vi "data更新获取索引操作函数.vi"(8 "error in (no error)":errorcluster, 9 "当前操作行":i32, 10 "当前_datetime":string, 11 "缓存操作选项":T1) -> (0 "error out":errorcluster, 3 "Data_CT索引操作缓存":T2)   [LabVIEW 2017]
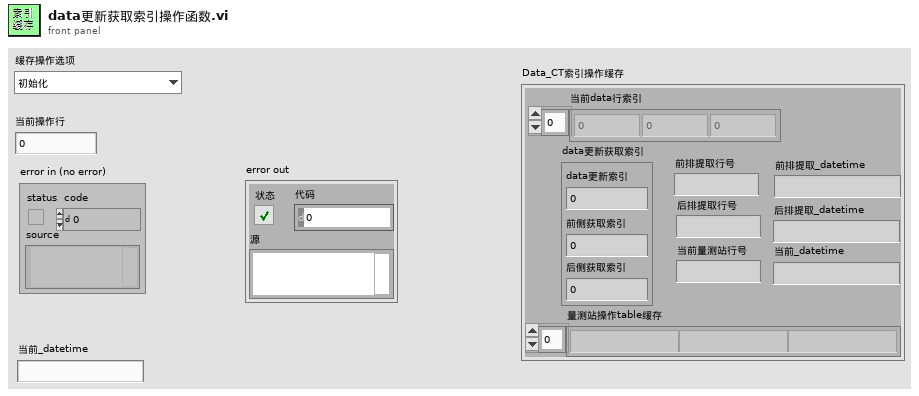
[diagram p1: front panel]
types:
  T1 = typedef "缓存操作选项.ctl" = enum16{"初始化", "量测缓存写入", "前侧获取索引", "后侧获取索引", "前侧更新索引", "后侧更新索引", "获取寄存器"}
  T2 = typedef "Data_CT索引操作缓存.ctl" = cluster{"当前data行索引":i32[], "data更新获取索引":T3, "前排提取行号":string, "后排提取行号":string, "当前量测站行号":string, "当前_datetime":string, "量测站操作table缓存":string[], "前排提取_datetime":string, "后排提取_datetime":string}
  T3 = typedef "data更新获取索引.ctl" = cluster{"data更新索引":i32, "前侧获取索引":i32, "后侧获取索引":i32}
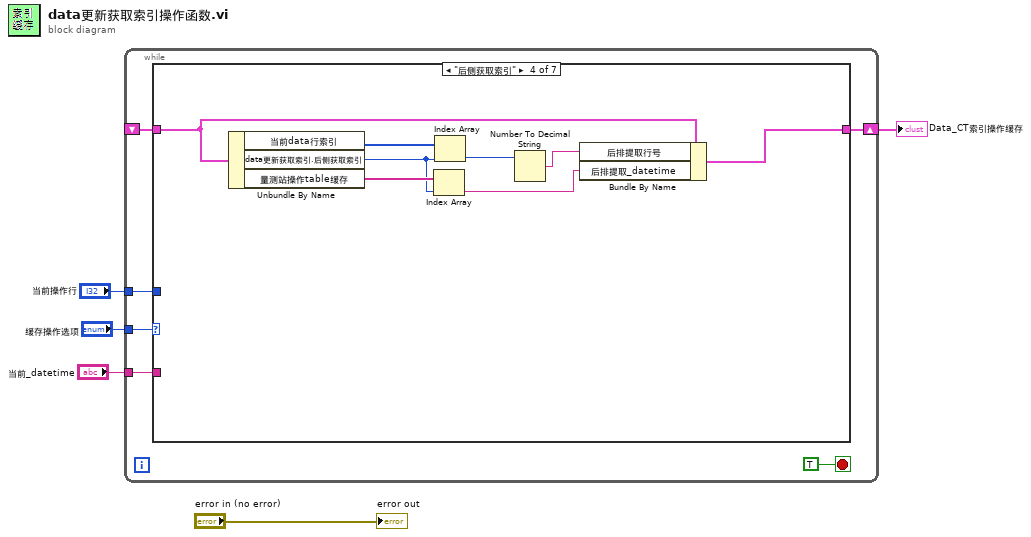
[diagram p0: block diagram]
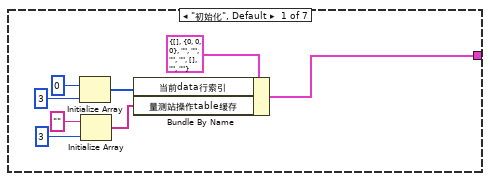
[diagram p2: hidden frame]
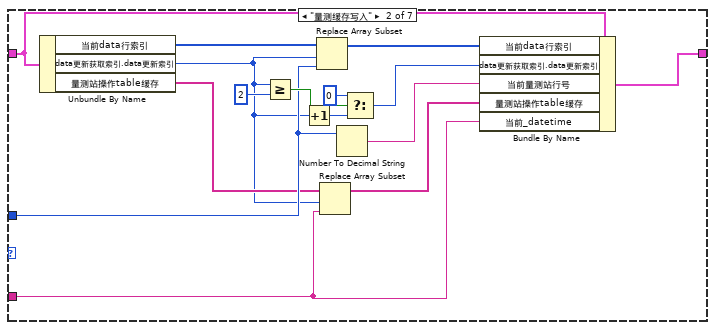
[diagram p3: hidden frame]
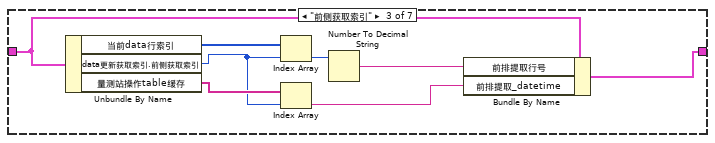
[diagram p4: hidden frame]
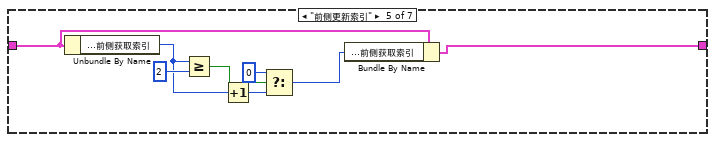
[diagram p5: hidden frame]
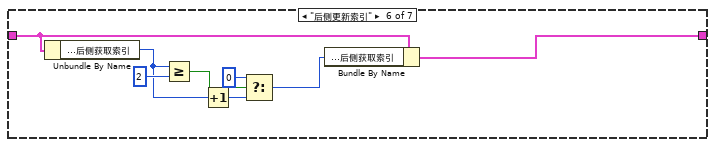
[diagram p6: hidden frame]
diagram:
  n1 = while {
    tunnel: "缓存操作选项" -> [w11]
    shift-right: [w9] -> w4
    shift-left: _ -> [w8]
    tunnel: "当前操作行" -> [w7]
    tunnel: "当前_datetime" -> [w6]
    stop <- TRUE stop-if-true
    n2 = case shown="\"后侧获取索引\"" w11 {
      tunnel: [w18 w31 w38 w46 w51 w59 w67] -> w9
      tunnel: w8 -> [_ w33 w41 w47 w53 w60 w67]
      tunnel: w7 -> [_ w25 _ _ _ _ _]
      tunnel: w6 -> [_ w20 _ _ _ _ _]
      frame "初始化", Default {
        n3 = Initialize Array(0, 3 ("维数大小")) -> (w15:i32[])
        n4 = Initialize Array("", 3 ("维数大小")) -> (w13:string[])
        n5 = Bundle By Name(cluster=T2 {"当前data行索引"=[], "data更新获取索引"={"data更新索引"=0, "前侧获取索引"=0, "后侧获取索引"=0}, "前排提取行号"="", "后排提取行号"="", "当前量测站行号"="", "当前_datetime"="", "量测站操作table缓存"=[], "前排提取_datetime"="", "后排提取_datetime"=""} ("Data_CT索引操作缓存"), "当前data行索引"=w15, "量测站操作table缓存"=w13) -> (w18:T2)
      }
      frame "量测缓存写入" {
        n6 = Unbundle By Name(w33) -> ("当前data行索引"=w34:i32[], "data更新获取索引.data更新索引"=w22:i32, "量测站操作table缓存"=w23:string[])
        n7 = Greater Or Equal?(x=w22, y=2) -> (x >= y?=w29:bool)
        n8 = Increment(x=w22) -> (x+1=w28:i32)
        n9 = Replace Array Subset(array=w34, new element=w25, index=w22) -> (w32:i32[])
        n10 = Replace Array Subset(array=w23, new element=w20, index=w22) -> (w21:string[])
        n11 = Number To Decimal String(number=w25) -> (decimal integer string=w24:string)  [unwired: 1 in]
        n12 = Select(t=0 ("y"), s=w29, f=w28) -> (s? t:f=w26:i32)
        n13 = Bundle By Name(cluster=w33, "当前data行索引"=w32, "data更新获取索引.data更新索引"=w26, "当前量测站行号"=w24, "量测站操作table缓存"=w21, "当前_datetime"=w20) -> (w31:T2)
      }
      frame "前侧获取索引" {
        n14 = Unbundle By Name(w41) -> ("当前data行索引"=w42:i32[], "data更新获取索引.前侧获取索引"=w36:i32, "量测站操作table缓存"=w37:string[])
        n15 = Index Array(array=w42, index=w36) -> (element=w40:i32)
        n16 = Index Array(array=w37, index=w36) -> (element=w35:string)
        n17 = Number To Decimal String(number=w40) -> (decimal integer string=w39:string)  [unwired: 1 in]
        n18 = Bundle By Name(cluster=w41, "前排提取行号"=w39, "前排提取_datetime"=w35) -> (w38:T2)
      }
      frame "后侧获取索引" {
        n19 = Unbundle By Name(w47) -> ("当前data行索引"=w50:i32[], "data更新获取索引.后侧获取索引"=w44:i32, "量测站操作table缓存"=w45:string[])
        n20 = Index Array(array=w45, index=w44) -> (element=w43:string)
        n21 = Index Array(array=w50, index=w44) -> (element=w49:i32)
        n22 = Number To Decimal String(number=w49) -> (decimal integer string=w48:string)  [unwired: 1 in]
        n23 = Bundle By Name(cluster=w47, "后排提取行号"=w48, "后排提取_datetime"=w43) -> (w46:T2)
      }
      frame "前侧更新索引" {
        n24 = Unbundle By Name(w53) -> ("data更新获取索引.前侧获取索引"=w54:i32)
        n25 = Greater Or Equal?(x=w54, y=2) -> (x >= y?=w57:bool)
        n26 = Increment(x=w54) -> (x+1=w56:i32)
        n27 = Select(t=0 ("y"), s=w57, f=w56) -> (s? t:f=w52:i32)
        n28 = Bundle By Name(cluster=w53, "data更新获取索引.前侧获取索引"=w52) -> (w51:T2)
      }
      frame "后侧更新索引" {
        n29 = Unbundle By Name(w60) -> ("data更新获取索引.后侧获取索引"=w62:i32)
        n30 = Greater Or Equal?(x=w62, y=2) -> (x >= y?=w65:bool)
        n31 = Increment(x=w62) -> (x+1=w64:i32)
        n32 = Select(t=0 ("y"), s=w65, f=w64) -> (s? t:f=w61:i32)
        n33 = Bundle By Name(cluster=w60, "data更新获取索引.后侧获取索引"=w61) -> (w59:T2)
      }
      frame "获取寄存器" {
      }
    }
  }
  "Data_CT索引操作缓存" <- w4
  "error out" <- "error in (no error)"
